vi "Power interface Check if Unipower.vi"(0 "VISA Refnum in":refnum<visa-resource-name>, 11 "error in (no error)":errorcluster) -> (8 "PSU type":T1, 13 "Found PSU":bool, 15 "error out":errorcluster)   [LabVIEW 2011]
uses:
  PCP interface/PSU Type.ctl
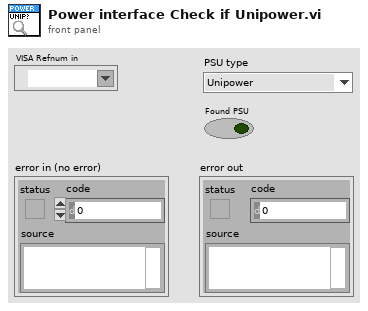
[diagram p1: front panel]
types:
  T1 = typedef "PSU Type.ctl" = enum16{"Unipower", "Magna 8.3A", "Magna 12A", "None"}
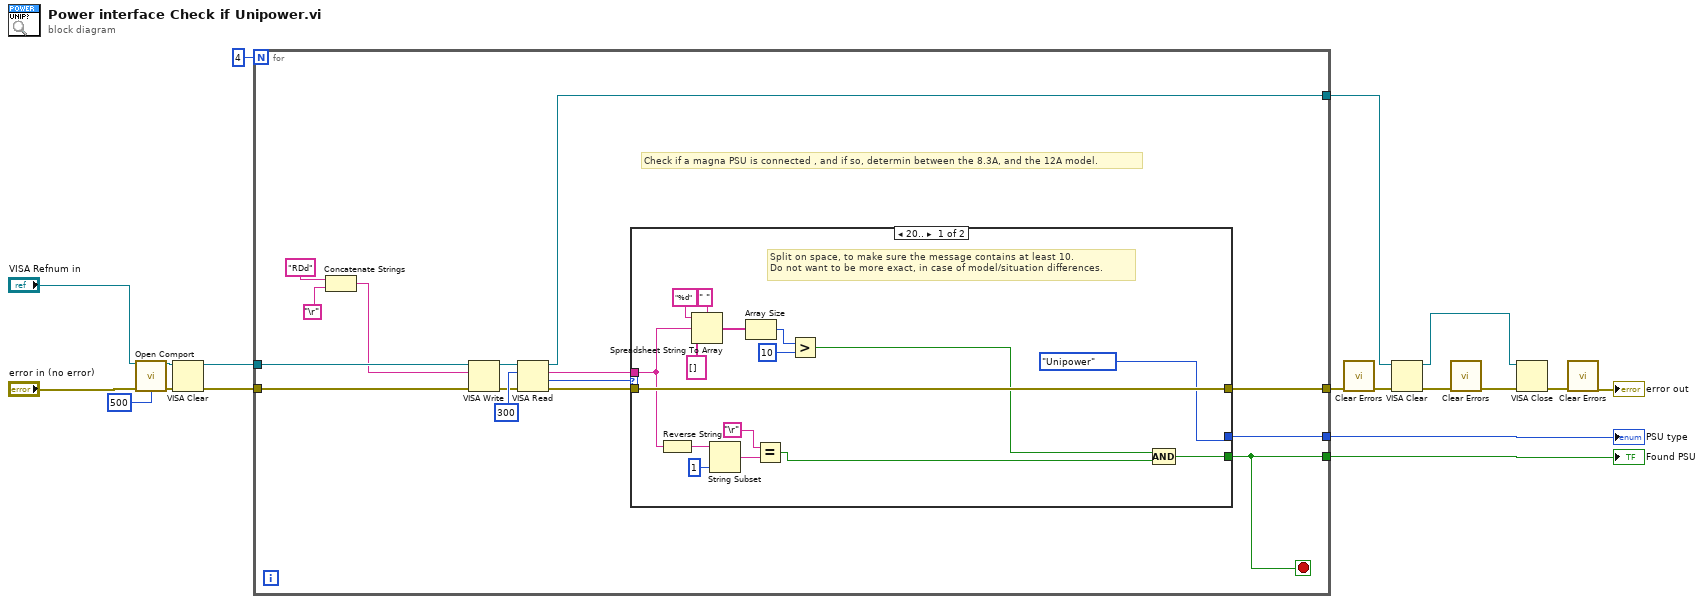
[diagram p0: block diagram]
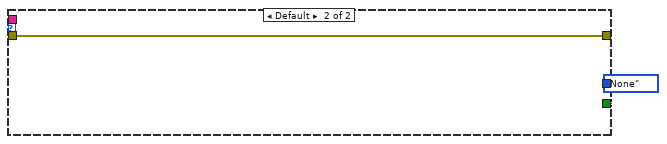
[diagram p2: hidden frame]
diagram:
  n1 = call "Open Comport.vi"("Comport"="VISA Refnum in", "error in (no error)"="error in (no error)", "Reply timeout (300 ms)"=u32 500) -> ("VISA resource name out"=w7:refnum<visa-resource-name>, "error out"=w9:errorcluster)  [unwired: 11 in]
  n2 = VISA Clear(VISA resource name=w7, error in (no error)=w9) -> (VISA resource name out=w16:refnum<visa-resource-name>, error out=w15:errorcluster)
  n3 = for {
    N: 4 -> [_]
    tunnel: [w33] -> w18
    tunnel: [w19] -> w17
    tunnel: w16 -> [w26]
    tunnel: w15 -> [w25]
    tunnel: [w24] -> w14
    tunnel: [w23] -> w13
    stop <- w19 stop-if-true
    # "Check if a magna PSU is connected , and if so, determin between the 8.3A, and the 12A model."
    n4 = Concatenate Strings("RDd", "\r") -> (w20:string)
    n5 = VISA Write(VISA resource name=w26, write buffer=w20, error in (no error)=w25) -> (VISA resource name out=w28:refnum<visa-resource-name>, error out=w27:errorcluster)  [unwired: 1 out]
    n6 = VISA Read(VISA resource name=w28, byte count=u32 300, error in (no error)=w27) -> (VISA resource name out=w23:refnum<visa-resource-name>, read buffer=w32:string, return count=w30:u32, error out=w31:errorcluster)
    n7 = case shown="20.." w30 {
      tunnel: w31 -> [w46 w52]
      tunnel: [w46 w52] -> w24
      tunnel: w32 -> [w43 _]
      tunnel: [w45 FALSE] -> w19
      tunnel: [PSU_Type."Unipower" ("PSU type") PSU_Type."None" ("PSU type")] -> w33
      frame 20.. {
        # "Split on space, to make sure the message contains at least 10.\nDo not want to be more exact, in case of model/situation differences."
        n8 = Reverse String(1:w43) -> (0:w42:string)
        n9 = Spreadsheet String To Array(delimiter (Tab)=" ", format string="%d", spreadsheet string=w43, array type (2D Dbl)=string[] []) -> (array=w38:string[])
        n10 = String Subset(string=w42, length (rest)=1 ("length (rest)")) -> (substring=w40:string)  [unwired: 1 in]
        n11 = Array Size(array=w38) -> (size(s)=w37:i32)
        n12 = Equal?(x="\r", y=w40) -> (x = y?=w34:bool)
        n13 = Greater?(x=w37, y=10) -> (0:w35:bool)
        n14 = Compound Arithmetic op=AND(w35, w34) -> (w45:bool)
      }
      frame Default {
      }
    }
  }
  "PSU type" <- w18
  "Found PSU" <- w17
  n15 = call <vilib>:"Clear Errors.vi"("error in (no error)"=w14) -> ("error out"=w5:errorcluster)  [unwired: 6 in]
  n16 = VISA Clear(VISA resource name=w13, error in (no error)=w5) -> (VISA resource name out=w4:refnum<visa-resource-name>, error out=w3:errorcluster)
  n17 = call <vilib>:"Clear Errors.vi"("error in (no error)"=w3) -> ("error out"=w2:errorcluster)  [unwired: 6 in]
  n18 = VISA Close(VISA resource name=w4, error in (no error)=w2) -> (error out=w11:errorcluster)
  n19 = call <vilib>:"Clear Errors.vi"("error in (no error)"=w11) -> ("error out"=→"error out":errorcluster)  [unwired: 6 in]
